vi "Round To Nearest Increment.vi"(10 "Increments to round":dbl=100.0, 11 "Number":dbl=240.0) -> (3 "Rounded Number":dbl)   [LabVIEW 2015]
doc: "This VI will round <b>Number</b> the the increment in <b>Increment to round</b> and return it on <b>Rounded Number</b>."
panel:
  # "`"
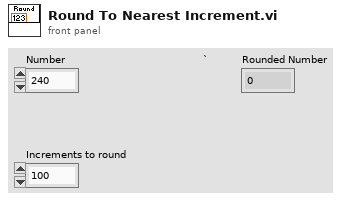
[diagram p1: front panel]
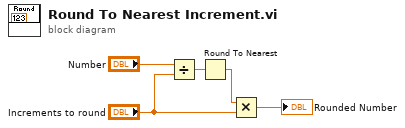
[diagram p0: block diagram]
diagram:
  n1 = Divide(x="Number", y="Increments to round") -> (x/y=w5:dbl)
  n2 = Round To Nearest(number=w5) -> (nearest integer value=w1:dbl)
  n3 = Multiply(x=w1, y="Increments to round") -> (x*y=→"Rounded Number":dbl)
